vi "Global 2.vi"() -> ()   [LabVIEW 2014]
panel:
  in  "Forklift Out":bool
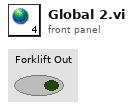
[diagram p1: front panel]
diagram:
